vi "List Devices Example.vi"() -> ()   [LabVIEW 2019, in "D2XX-lv.lvlib"]
uses:
  D2XX-lv.lvlib
  typedefs/Device Info.ctl
panel:
  in  "Filter (Device Description)":string="7008"
  out "Devices":T1[](array[typedef])
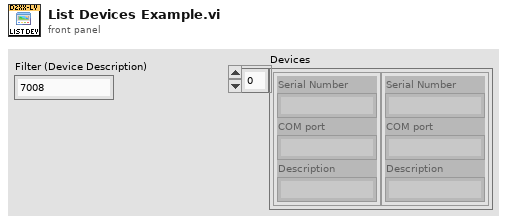
[diagram p1: front panel]
types:
  T1 = typedef "D2XX-lv.lvlib/Device Info.ctl" = cluster{"Serial Number":string, "COM port":string, "Description":string}
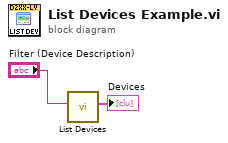
[diagram p0: block diagram]
diagram:
  n1 = call "List Devices.vi"("Filter (Device Description)"="Filter (Device Description)") -> ("Devices"=→"Devices":T1[])  [unwired: 9 in, 1 out]
